vi "GetMetadataKey.vi"(8 "error in (no error)":errorcluster, 10 "index":i32, 11 "session id in":i32) -> (0 "error out":errorcluster, 1 "MetadataKey":string, 2 "GetMetadataKey":bool, 3 "session id out":i32)   [LabVIEW 2017, in "libonnx_wrapper.lvlib"]
doc: "/**\n * @brief Получить ключ метаданных по индексу\n * \n * @param sessionId [IN] ID сессии\n * @param index [IN] Индекс метаданных (0-based)\n * @param buffer [OUT] Буфер для строки с ключом\n * @param bufferSize [IN] Размер буфера (рекомендуется 256)\n * \n * @return int32: 0 при успехе\n * @return int32: -1 если индекс неверен\n * \n * @example Ключи: \"producer_name\", \"graph_name\", \"model_version\"\n */\nint GetMetadataKey(int sessionId, int index, char* buffer, int bufferSize);"
uses:
  libonnx_wrapper.lvlib
panel:
  out "bufferSize":i32
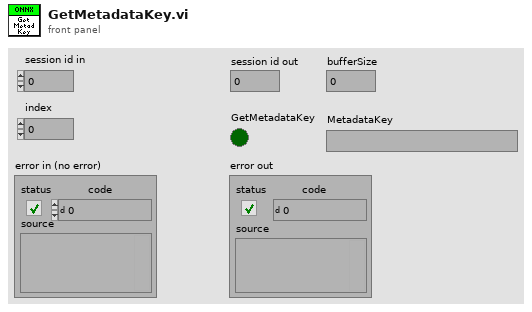
[diagram p1: front panel]
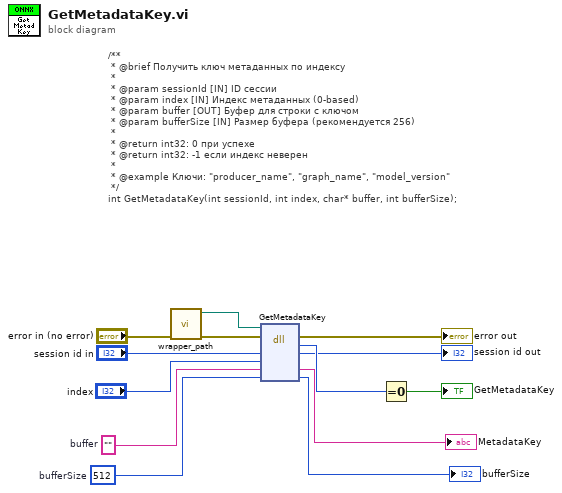
[diagram p0: block diagram]
diagram:
  w9 = 512  # bufferSize
  w11 = ""  # buffer
  # "/**\n * @brief Получить ключ метаданных по индексу\n * \n * @param sessionId [IN] ID сессии\n * @param index [IN] Индекс метаданных (0-based)\n * @param buffer [OUT] Буфер для строки с ключом\n * @param bufferSize [IN] Размер буфера (рекомендуется 256)\n * \n * @return int32: 0 при успехе\n * @return int32: -1 если индекс неверен\n * \n * @example Ключи: \"producer_name\", \"graph_name\", \"model_version\"\n */\nint GetMetadataKey(int sessionId, int index, char* buffer, int bufferSize);"
  n1 = call "wrapper_path.vi"("error in (no error)"="error in (no error)") -> ("error out"=w4:errorcluster, "wrapper path"=w7:path)  [unwired: 9 in]
  n2 = dll-call lib="home/ivan/LabVIEWData/ONNX/Test/libonnx_wrapper/unix64/libonnx_wrapper.so" fn="GetMetadataKey"(path in=w7, error in=w4, "sessionId"="session id in", "inputIndex"="index", "buffer"=w11, "bufferSize"=w9) -> (error out=→"error out":errorcluster, "GetMetadataKey"=w13:i32, "sessionId"=→"session id out":i32, "buffer"=→"MetadataKey":string, "bufferSize"=→"bufferSize":i32)  [unwired: 2 in, 1 out]
  n3 = Equal To 0?(x=w13) -> (x = 0?=→"GetMetadataKey":bool)
